vi "Close_Loop_Motor_Tune.vi"() -> ()   [LabVIEW 2019]
uses:
  <vilib>/rvi/Emulation/niFpgaGetClockAttributes.vi
  <vilib>/rvi/Emulation/niFpgaSctlEmulationGetInTimedLoop.vi
  <vilib>/rvi/Emulation/niFpgaEmulationReportErrorSimple.vi
  <vilib>/rvi/eio/common/nirviEmuTemplateMethod_errors.vi
  <vilib>/rvi/Emulation/niFpgaCriticalErrorInLSC.vi
  <vilib>/eio/EIONode/EIONode.xnode
  <vilib>/rvi/Arithmetic/AddSubMult/XNode/nirviSatArithmetic.xnode
panel:
  in  "Motor3_KP":sgl
  in  "Motor2_KP":sgl
  in  "Motor1_KP":sgl=1.2
  in  "Position Reset 3":bool
  out "Position (Counts) motor side 3":i16
  out "Acceleration (Counts/Interval) motor side 3":i32
  out "Velocity (Counts/Interval) motor side 3":i32
  out "Loop time (position) 1 motor side 3":u32
  out "Position(Radians) motor side 3":sgl(graph)
  out "Boolean 4":bool
  in  "desired angle 3":sgl
  in  "Position Reset 2":bool
  out "Position (Counts) motor side 2":i16
  out "Acceleration (Counts/Interval) motor side 2":i32
  out "Velocity (Counts/Interval) motor side 2":i32
  out "Loop time (position) 1 motor side 2":u32
  out "Position(Radians) motor side 2":sgl(graph)
  out "Boolean 3":bool
  in  "desired angle 2":sgl
  in  "Position Reset":bool
  out "Position (Counts) motor side":i16
  out "Acceleration (Counts/Interval) motor side":i32
  out "Velocity (Counts/Interval) motor side":i32
  out "Loop time (position) 1 motor side":u32
  out "Position(Radians) motor side":sgl(graph)
  out "Boolean 2":bool
  in  "desired angle":sgl
  out "duty cycle":sgl
  in  "Position Reset 2_e":bool
  out "Position (Counts) motor side 2_e":i16
  out "Acceleration (Counts/Interval) motor side 2_e":i32
  out "Velocity (Counts/Interval) motor side 2_e":i32
  out "Loop time (position) 1 motor side 2_e":u32
  out "Position(Radians) motor side 2_e":sgl(graph)
  out "Boolean 3_e":bool
  in  "desired angle 2(error)":sgl
  in  "Position Reset 3_e":bool
  out "Position (Counts) motor side 3_e":i16
  out "Acceleration (Counts/Interval) motor side 3_e":i32
  out "Velocity (Counts/Interval) motor side 3_e":i32
  out "Loop time (position) 1 motor side 3_e":u32
  out "Position(Radians) motor side 3_e":sgl(graph)
  out "Boolean 4_e":bool
  in  "desired angle 3(error)":sgl
  in  "Position Reset_e":bool
  out "Position (Counts) motor side_e":i16
  out "Acceleration (Counts/Interval) motor side_e":i32
  out "Velocity (Counts/Interval) motor side_e":i32
  out "Loop time (position) 1 motor side _e":u32
  out "Position(Radians) motor side_e":sgl(graph)
  out "Boolean 2_e":bool
  in  "desired angle (error)":sgl
  out "duty cycle 1_e":sgl
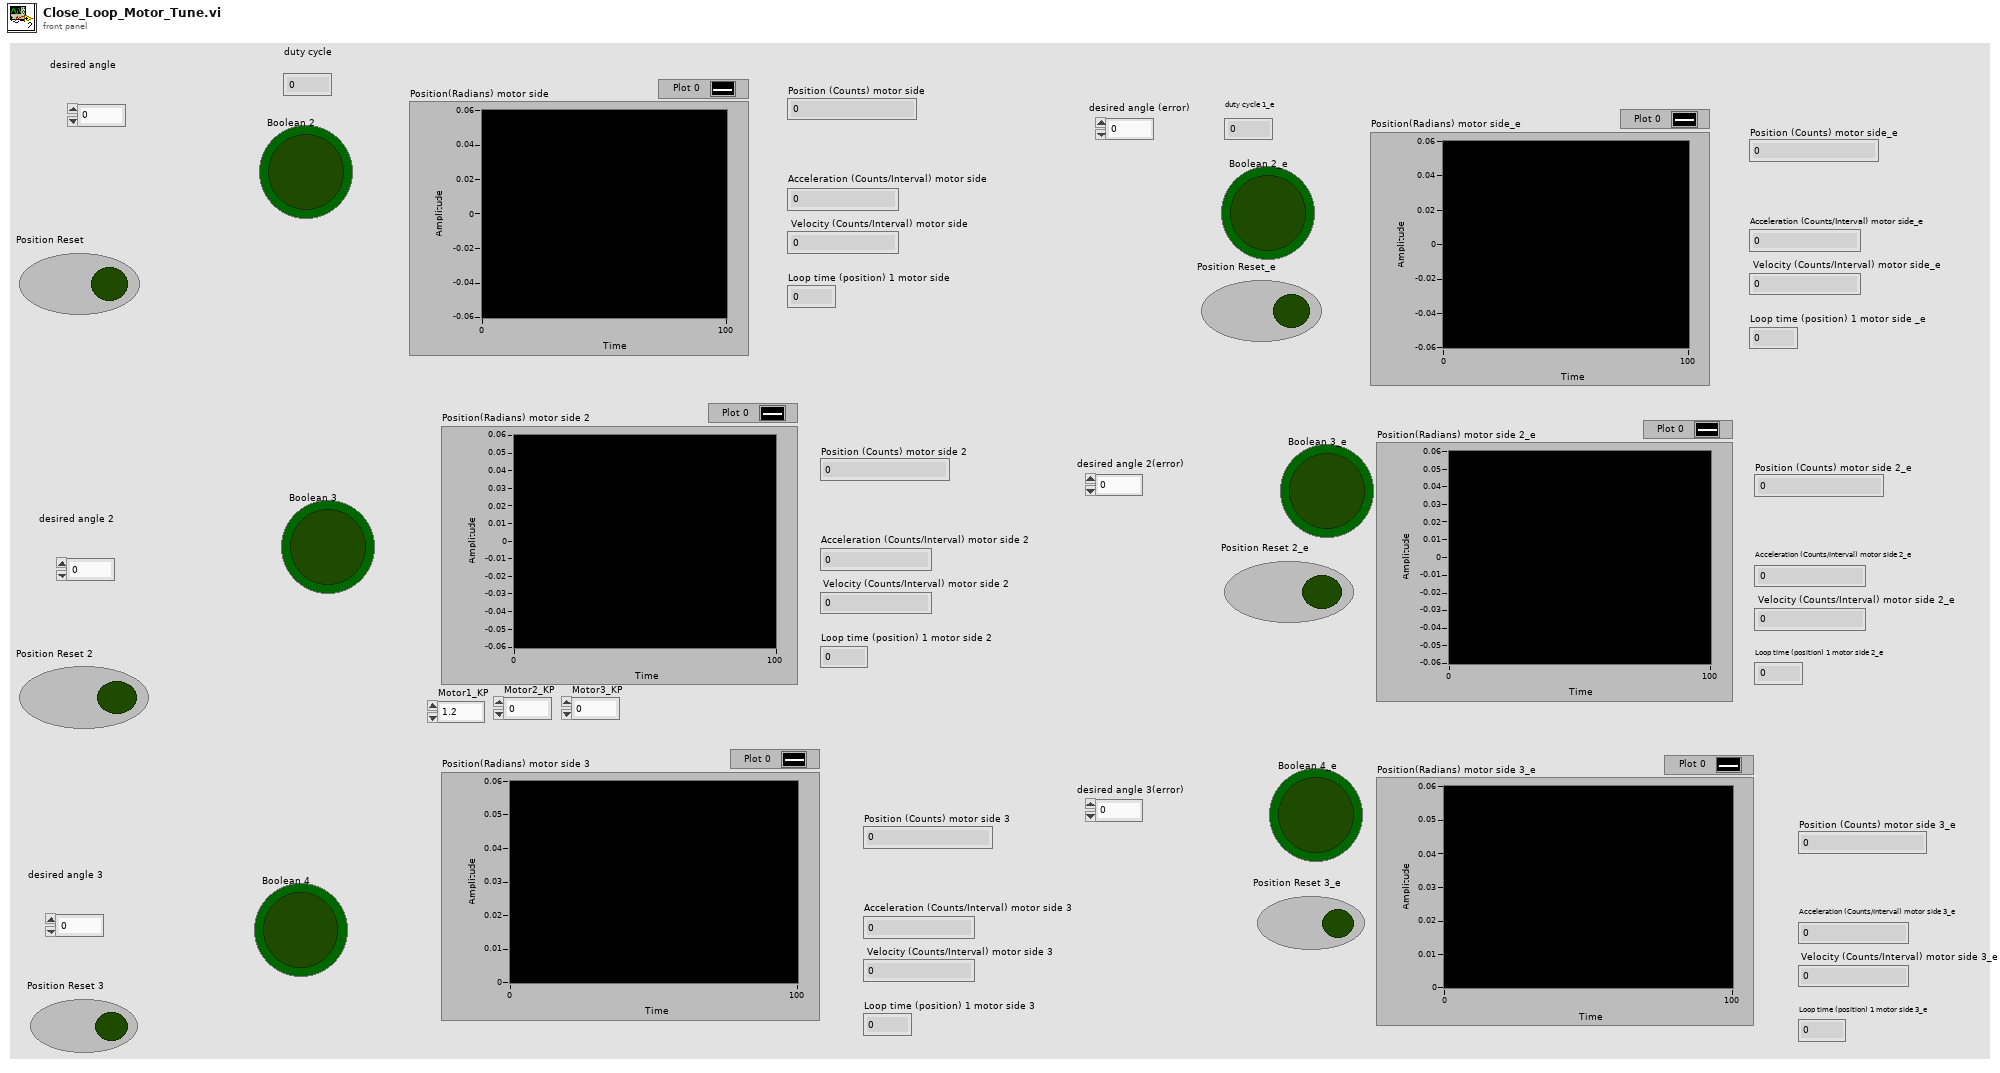
[diagram p1: front panel]
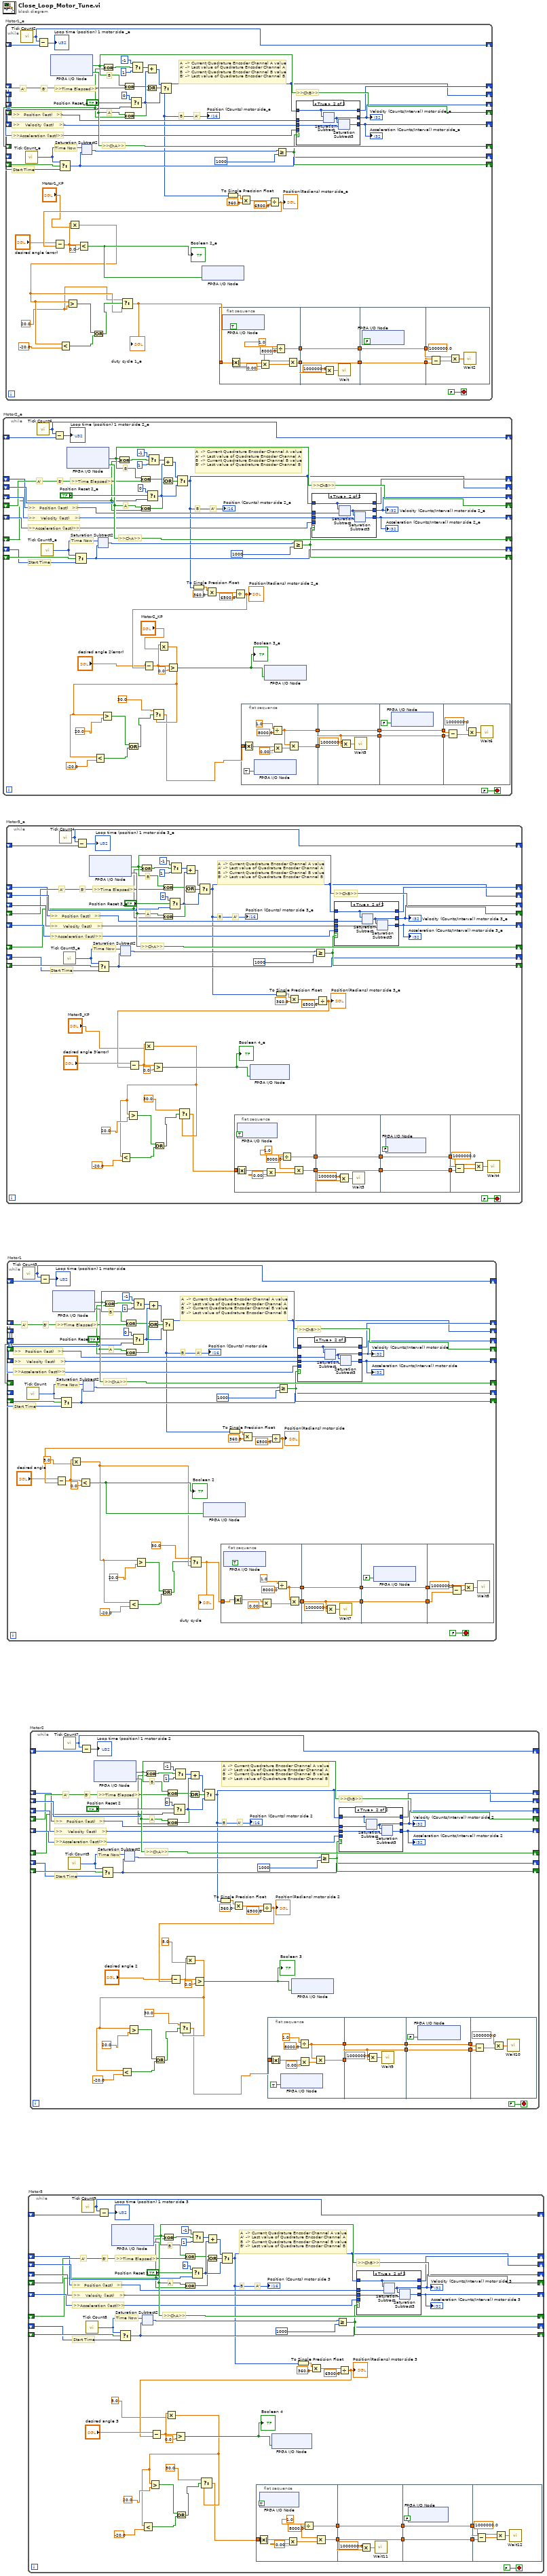
[diagram p0: block diagram]
diagram:
  n1 = while "Motor2_e" {
    shift-right: [w48] -> _
    shift-left: _ -> [w36]
    shift-right: [w28] -> _
    shift-left: _ -> [w45]
    shift-right: [w47] -> _
    shift-left: _ -> [w10]
    shift-right: [w42] -> _
    shift-left: _ -> [w44]
    shift-right: [w38] -> _
    shift-left: _ -> [w43]
    shift-right: [w33] -> _
    shift-left: _ -> [w32]
    shift-right: [w34] -> _
    shift-left: _ -> [w40]
    shift-right: [w35] -> _
    shift-left: _ -> [w37]
    shift-right: [w29] -> _
    shift-left: _ -> [w31]
    stop <- FALSE stop-if-true
    # "A  -> Current Quadrature Encoder Channel A value\nA' -> Last value of Quadrature Encoder Channel A\nB  -> Current Quadrature Encoder Channel B value\nB' -> Last value of Quadrature Encoder Channel B"
    # ">>Acceleration (last)>>"
    # "Start Time"
    # "A'"
    # "B"
    # "A'"
    # "A"
    # "B'"
    # "B"
    # ">>ChB>>"
    # ">>ChA>>"
    # ">>    Velocity (last)    >>"
    # ">>   Position (last)   >>"
    # "Time Now"
    # ">>Time Elapsed>>"
    n2 = call "Tick Count6"() -> ("Tick Count(Ticks)"=w29:u32)
    n3 = call "Tick Count5_e"() -> ("Tick Count(uSec)"=w39:u32)
    n4 = Subtract(x=w29, y=w31) -> (x-y=→"Loop time (position) 1 motor side 2_e":u32)
    n5 = xnode "FPGA I/O Node"() -> ("RMC/DIO12"=w48:bool, "RMC/DIO13"=w47:bool)  [unwired: 2 in, 2 out]
    n6 = Select(t=w39, s=w44, f=w43) -> (s? t:f=w38:u32)
    n7 = xnode ("Saturation Subtract2")("x"=w39, "y"=w38) -> ("x-y"=w41:u32)
    n8 = Exclusive Or(1:w10, 2:w48) -> (0:w49:bool)
    n9 = Exclusive Or(1:w36, 2:w48) -> (0:w50:bool)
    n10 = Exclusive Or(1:w10, 2:w47) -> (0:w51:bool)
    n11 = Select(t=0 ("32 bit"), s="Position Reset 2_e", f=w45) -> (s? t:f=w56:i32)
    n12 = Select(t=-1 ("32 bit"), s=w49, f=1 ("32 bit")) -> (s? t:f=w54:i32)
    n13 = Add(x=w54, y=w56) -> (x+y=w58:i32)
    n14 = Or(x=w50, y=w51) -> (x .or. y?=w46:bool)
    n15 = Select(t=w58, s=w46, f=w56) -> (s? t:f=w28:i32)
    "Position (Counts) motor side 2_e" <- w28
    n16 = To Single Precision Float(number=w28) -> (single precision float=w27:sgl)
    n17 = Multiply(x=w27, y=sgl 360.0) -> (x*y=w26:sgl)
    n18 = Divide(x=w26, y=sgl 6500.0) -> (x/y=w15:sgl)
    "Position(Radians) motor side 2_e" <- w15
    n19 = Subtract(x="desired angle 2(error)", y=w15) -> (x-y=w14:sgl)
    n20 = Multiply(x=w14, y="Motor2_KP") -> (x*y=w3:sgl)
    n21 = Less?(x=w3, y=sgl -20.0) -> (x < y?=w9:bool)
    n22 = Greater?(x=w3, y=sgl 20.0 ("constrain max")) -> (0:w8:bool)
    n23 = Or(x=w8, y=w9) -> (x .or. y?=w5:bool)
    n24 = Select(t=sgl 30.0 ("kp1"), s=w5, f=w3) -> (s? t:f=w2:sgl)
    n25 = Greater?(x=w14, y=sgl 0.0) -> (0:w12:bool)
    "Boolean 3_e" <- w12
    n26 = flat-sequence {
      tunnel: [w64] -> w22
      tunnel: [w62] -> w21
      tunnel: w2 -> [w60]
      tunnel: w22 -> [w69]
      tunnel: [w69] -> w20
      tunnel: w21 -> [w68]
      tunnel: [w68] -> w19
      tunnel: w20 -> [w74]
      tunnel: [w74] -> w18
      tunnel: w19 -> [w73]
      tunnel: [w73] -> w17
      tunnel: w18 -> [w79]
      tunnel: w17 -> [w75]
      frame #0 {
        n27 = Absolute Value(x=w60) -> (abs(x)=w59:sgl)
        n28 = xnode "FPGA I/O Node"("RMC/DIO16"=TRUE) -> ()  [unwired: 1 in, 1 out]
        n29 = Divide(x=sgl 1.0, y=sgl 8000.0) -> (x/y=w62:sgl)
        n30 = Multiply(x=w59, y=sgl 0.01) -> (x*y=w65:sgl)
        n31 = Multiply(x=w62, y=w65) -> (x*y=w64:sgl)
      }
      frame #1 {
        n32 = Multiply(x=sgl 1000000.0, y=w69) -> (x*y=w71:sgl)
        n33 = call "Wait5"("Count(uSec)"=w71) -> ()  [unwired: 1 out]
      }
      frame #2 {
        n34 = xnode "FPGA I/O Node"("RMC/DIO16"=FALSE) -> ()  [unwired: 1 in, 1 out]
      }
      frame #3 {
        n35 = Subtract(x=w75, y=w79) -> (x-y=w78:sgl)
        n36 = Multiply(x=sgl 1000000.0, y=w78) -> (x*y=w77:sgl)
        n37 = call "Wait6"("Count(uSec)"=w77) -> ()  [unwired: 1 out]
      }
    }
    n38 = xnode "FPGA I/O Node"("RMC/DIO17"=w12) -> ()  [unwired: 1 in, 1 out]
    n39 = Greater Or Equal?(x=w41, y=u32 1000) -> (x >= y?=w42:bool)
    n40 = case shown="True" w42 {
      tunnel: w28 -> [_ w93]
      tunnel: w32 -> [w90 w97]
      tunnel: [w92 w96] -> w34
      tunnel: w40 -> [w92 w95]
      tunnel: [w91 w94] -> w35
      tunnel: w37 -> [w91 _]
      tunnel: [w90 w93] -> w33
      frame False {
      }
      frame True {
        n41 = xnode ("Saturation Subtract")("x"=w93, "y"=w97) -> ("x-y"=w96:i32)
        n42 = xnode ("Saturation Subtract3")("x"=w96, "y"=w95) -> ("x-y"=w94:i32)
      }
    }
    "Acceleration (Counts/Interval) motor side 2_e" <- w35
    "Velocity (Counts/Interval) motor side 2_e" <- w34
  }
  n43 = while "Motor1_e" {
    shift-right: [w180] -> _
    shift-left: _ -> [w168]
    shift-right: [w159] -> _
    shift-left: _ -> [w177]
    shift-right: [w179] -> _
    shift-left: _ -> [w160]
    shift-right: [w174] -> _
    shift-left: _ -> [w176]
    shift-right: [w170] -> _
    shift-left: _ -> [w175]
    shift-right: [w165] -> _
    shift-left: _ -> [w164]
    shift-right: [w166] -> _
    shift-left: _ -> [w172]
    shift-right: [w167] -> _
    shift-left: _ -> [w169]
    shift-right: [w161] -> _
    shift-left: _ -> [w163]
    stop <- FALSE stop-if-true
    w136 = sgl 20.0 ("constrain max")
    # "A  -> Current Quadrature Encoder Channel A value\nA' -> Last value of Quadrature Encoder Channel A\nB  -> Current Quadrature Encoder Channel B value\nB' -> Last value of Quadrature Encoder Channel B"
    # ">>Acceleration (last)>>"
    # "Start Time"
    # "A'"
    # "B"
    # "A'"
    # "A"
    # "B'"
    # "B"
    # ">>ChB>>"
    # ">>ChA>>"
    # ">>    Velocity (last)    >>"
    # ">>   Position (last)   >>"
    # "Time Now"
    # ">>Time Elapsed>>"
    n44 = call "Tick Count2"() -> ("Tick Count(Ticks)"=w161:u32)
    n45 = call "Tick Count_e"() -> ("Tick Count(uSec)"=w171:u32)
    n46 = Subtract(x=w161, y=w163) -> (x-y=→"Loop time (position) 1 motor side _e":u32)
    n47 = xnode "FPGA I/O Node"() -> ("RMC/DIO45"=w180:bool, "RMC/DIO43"=w179:bool)  [unwired: 2 in, 2 out]
    n48 = Select(t=w171, s=w176, f=w175) -> (s? t:f=w170:u32)
    n49 = xnode ("Saturation Subtract2")("x"=w171, "y"=w170) -> ("x-y"=w173:u32)
    n50 = Exclusive Or(1:w160, 2:w180) -> (0:w181:bool)
    n51 = Exclusive Or(1:w168, 2:w180) -> (0:w182:bool)
    n52 = Exclusive Or(1:w160, 2:w179) -> (0:w183:bool)
    n53 = Select(t=0 ("32 bit"), s="Position Reset_e", f=w177) -> (s? t:f=w188:i32)
    n54 = Select(t=-1 ("32 bit"), s=w181, f=1 ("32 bit")) -> (s? t:f=w186:i32)
    n55 = Add(x=w186, y=w188) -> (x+y=w190:i32)
    n56 = Or(x=w182, y=w183) -> (x .or. y?=w178:bool)
    n57 = Select(t=w190, s=w178, f=w188) -> (s? t:f=w159:i32)
    "Position (Counts) motor side_e" <- w159
    n58 = flat-sequence {
      tunnel: [w196] -> w153
      tunnel: [w194] -> w152
      tunnel: w138 -> [w192]
      tunnel: w153 -> [w201]
      tunnel: [w201] -> w151
      tunnel: w152 -> [w200]
      tunnel: [w200] -> w150
      tunnel: w151 -> [w206]
      tunnel: [w206] -> w149
      tunnel: w150 -> [w205]
      tunnel: [w205] -> w148
      tunnel: w149 -> [w211]
      tunnel: w148 -> [w207]
      frame #0 {
        n59 = xnode "FPGA I/O Node"("RMC/DIO33"=TRUE) -> ()  [unwired: 1 in, 1 out]
        n60 = Absolute Value(x=w192) -> (abs(x)=w191:sgl)
        n61 = Multiply(x=w191, y=sgl 0.01) -> (x*y=w197:sgl)
        n62 = Divide(x=sgl 1.0, y=sgl 8000.0) -> (x/y=w194:sgl)
        n63 = Multiply(x=w194, y=w197) -> (x*y=w196:sgl)
      }
      frame #1 {
        n64 = Multiply(x=sgl 1000000.0, y=w201) -> (x*y=w203:sgl)
        n65 = call "Wait"("Count(uSec)"=w203) -> ()  [unwired: 1 out]
      }
      frame #2 {
        n66 = xnode "FPGA I/O Node"("RMC/DIO33"=FALSE) -> ()  [unwired: 1 in, 1 out]
      }
      frame #3 {
        n67 = Subtract(x=w207, y=w211) -> (x-y=w210:sgl)
        n68 = Multiply(x=sgl 1000000.0, y=w210) -> (x*y=w209:sgl)
        n69 = call "Wait2"("Count(uSec)"=w209) -> ()  [unwired: 1 out]
      }
    }
    n70 = To Single Precision Float(number=w159) -> (single precision float=w158:sgl)
    n71 = Multiply(x=w158, y=sgl 360.0) -> (x*y=w157:sgl)
    n72 = Divide(x=w157, y=sgl 6500.0) -> (x/y=w146:sgl)
    "Position(Radians) motor side_e" <- w146
    n73 = Subtract(x="desired angle (error)", y=w146) -> (x-y=w144:sgl)
    n74 = Multiply(x=w144, y="Motor1_KP") -> (x*y=w137:sgl)
    n75 = Less?(x=w137, y=sgl -20.0 ("constrain min")) -> (x < y?=w141:bool)
    n76 = Greater?(x=w137, y=w136) -> (0:w140:bool)
    n77 = Less?(x=w144, y=sgl 0.0) -> (x < y?=w143:bool)
    "Boolean 2_e" <- w143
    n78 = Or(x=w140, y=w141) -> (x .or. y?=w139:bool)
    n79 = Select(t=w136, s=w139, f=w137) -> (s? t:f=w138:sgl)
    "duty cycle 1_e" <- w138
    n80 = xnode "FPGA I/O Node"("RMC/DIO34"=w143) -> ()  [unwired: 1 in, 1 out]
    n81 = Greater Or Equal?(x=w173, y=u32 1000) -> (x >= y?=w174:bool)
    n82 = case shown="True" w174 {
      tunnel: w159 -> [_ w225]
      tunnel: w164 -> [w222 w229]
      tunnel: [w224 w228] -> w166
      tunnel: w172 -> [w224 w227]
      tunnel: [w223 w226] -> w167
      tunnel: w169 -> [w223 _]
      tunnel: [w222 w225] -> w165
      frame False {
      }
      frame True {
        n83 = xnode ("Saturation Subtract")("x"=w225, "y"=w229) -> ("x-y"=w228:i32)
        n84 = xnode ("Saturation Subtract3")("x"=w228, "y"=w227) -> ("x-y"=w226:i32)
      }
    }
    "Acceleration (Counts/Interval) motor side_e" <- w167
    "Velocity (Counts/Interval) motor side_e" <- w166
  }
  n85 = while "Motor3_e" {
    shift-right: [w313] -> _
    shift-left: _ -> [w301]
    shift-right: [w292] -> _
    shift-left: _ -> [w310]
    shift-right: [w312] -> _
    shift-left: _ -> [w293]
    shift-right: [w307] -> _
    shift-left: _ -> [w309]
    shift-right: [w303] -> _
    shift-left: _ -> [w308]
    shift-right: [w298] -> _
    shift-left: _ -> [w297]
    shift-right: [w299] -> _
    shift-left: _ -> [w305]
    shift-right: [w300] -> _
    shift-left: _ -> [w302]
    shift-right: [w294] -> _
    shift-left: _ -> [w296]
    stop <- FALSE stop-if-true
    # "A  -> Current Quadrature Encoder Channel A value\nA' -> Last value of Quadrature Encoder Channel A\nB  -> Current Quadrature Encoder Channel B value\nB' -> Last value of Quadrature Encoder Channel B"
    # ">>Acceleration (last)>>"
    # "Start Time"
    # "A'"
    # "B"
    # "A'"
    # "A"
    # "B'"
    # "B"
    # ">>ChB>>"
    # ">>ChA>>"
    # ">>    Velocity (last)    >>"
    # ">>   Position (last)   >>"
    # "Time Now"
    # ">>Time Elapsed>>"
    n86 = call "Tick Count4"() -> ("Tick Count(Ticks)"=w294:u32)
    n87 = call "Tick Count3_e"() -> ("Tick Count(uSec)"=w304:u32)
    n88 = Subtract(x=w294, y=w296) -> (x-y=→"Loop time (position) 1 motor side 3_e":u32)
    n89 = xnode "FPGA I/O Node"() -> ("RMC/DIO11"=w313:bool, "RMC/DIO10"=w312:bool)  [unwired: 2 in, 2 out]
    n90 = Select(t=w304, s=w309, f=w308) -> (s? t:f=w303:u32)
    n91 = xnode ("Saturation Subtract2")("x"=w304, "y"=w303) -> ("x-y"=w306:u32)
    n92 = Exclusive Or(1:w293, 2:w313) -> (0:w314:bool)
    n93 = Exclusive Or(1:w301, 2:w313) -> (0:w315:bool)
    n94 = Exclusive Or(1:w293, 2:w312) -> (0:w316:bool)
    n95 = Select(t=0 ("32 bit"), s="Position Reset 3_e", f=w310) -> (s? t:f=w321:i32)
    n96 = Select(t=-1 ("32 bit"), s=w314, f=1 ("32 bit")) -> (s? t:f=w319:i32)
    n97 = Add(x=w319, y=w321) -> (x+y=w323:i32)
    n98 = Or(x=w315, y=w316) -> (x .or. y?=w311:bool)
    n99 = Select(t=w323, s=w311, f=w321) -> (s? t:f=w292:i32)
    "Position (Counts) motor side 3_e" <- w292
    n100 = flat-sequence {
      tunnel: [w329] -> w286
      tunnel: [w327] -> w285
      tunnel: w268 -> [w325]
      tunnel: w286 -> [w334]
      tunnel: [w334] -> w284
      tunnel: w285 -> [w333]
      tunnel: [w333] -> w283
      tunnel: w284 -> [w339]
      tunnel: [w339] -> w282
      tunnel: w283 -> [w338]
      tunnel: [w338] -> w281
      tunnel: w282 -> [w344]
      tunnel: w281 -> [w340]
      frame #0 {
        n101 = Absolute Value(x=w325) -> (abs(x)=w324:sgl)
        n102 = xnode "FPGA I/O Node"("RMC/DIO0"=TRUE) -> ()  [unwired: 1 in, 1 out]
        n103 = Multiply(x=w324, y=sgl 0.01) -> (x*y=w330:sgl)
        n104 = Divide(x=sgl 1.0, y=sgl 8000.0) -> (x/y=w327:sgl)
        n105 = Multiply(x=w327, y=w330) -> (x*y=w329:sgl)
      }
      frame #1 {
        n106 = Multiply(x=sgl 1000000.0, y=w334) -> (x*y=w336:sgl)
        n107 = call "Wait3"("Count(uSec)"=w336) -> ()  [unwired: 1 out]
      }
      frame #2 {
        n108 = xnode "FPGA I/O Node"("RMC/DIO0"=FALSE) -> ()  [unwired: 1 in, 1 out]
      }
      frame #3 {
        n109 = Subtract(x=w340, y=w344) -> (x-y=w343:sgl)
        n110 = Multiply(x=sgl 1000000.0, y=w343) -> (x*y=w342:sgl)
        n111 = call "Wait4"("Count(uSec)"=w342) -> ()  [unwired: 1 out]
      }
    }
    n112 = To Single Precision Float(number=w292) -> (single precision float=w291:sgl)
    n113 = Multiply(x=w291, y=sgl 360.0) -> (x*y=w290:sgl)
    n114 = Greater Or Equal?(x=w306, y=u32 1000) -> (x >= y?=w307:bool)
    n115 = Divide(x=w290, y=sgl 6500.0) -> (x/y=w278:sgl)
    "Position(Radians) motor side 3_e" <- w278
    n116 = Subtract(x="desired angle 3(error)", y=w278) -> (x-y=w277:sgl)
    n117 = Multiply(x=w277, y="Motor3_KP") -> (x*y=w269:sgl)
    n118 = Less?(x=w269, y=sgl -20.0) -> (x < y?=w274:bool)
    n119 = Greater?(x=w269, y=sgl 20.0 ("constrain max")) -> (0:w273:bool)
    n120 = Greater?(x=w277, y=sgl 0.0) -> (0:w275:bool)
    "Boolean 4_e" <- w275
    n121 = Or(x=w273, y=w274) -> (x .or. y?=w270:bool)
    n122 = Select(t=sgl 30.0 ("kp1"), s=w270, f=w269) -> (s? t:f=w268:sgl)
    n123 = xnode "FPGA I/O Node"("RMC/DIO1"=w275) -> ()  [unwired: 1 in, 1 out]
    n124 = case shown="True" w307 {
      tunnel: w292 -> [_ w358]
      tunnel: w297 -> [w355 w362]
      tunnel: [w357 w361] -> w299
      tunnel: w305 -> [w357 w360]
      tunnel: [w356 w359] -> w300
      tunnel: w302 -> [w356 _]
      tunnel: [w355 w358] -> w298
      frame False {
      }
      frame True {
        n125 = xnode ("Saturation Subtract")("x"=w358, "y"=w362) -> ("x-y"=w361:i32)
        n126 = xnode ("Saturation Subtract3")("x"=w361, "y"=w360) -> ("x-y"=w359:i32)
      }
    }
    "Acceleration (Counts/Interval) motor side 3_e" <- w300
    "Velocity (Counts/Interval) motor side 3_e" <- w299
  }
  n127 = while "Motor1" {
    shift-right: [w446] -> _
    shift-left: _ -> [w434]
    shift-right: [w425] -> _
    shift-left: _ -> [w443]
    shift-right: [w445] -> _
    shift-left: _ -> [w426]
    shift-right: [w440] -> _
    shift-left: _ -> [w442]
    shift-right: [w436] -> _
    shift-left: _ -> [w441]
    shift-right: [w431] -> _
    shift-left: _ -> [w430]
    shift-right: [w432] -> _
    shift-left: _ -> [w438]
    shift-right: [w433] -> _
    shift-left: _ -> [w435]
    shift-right: [w427] -> _
    shift-left: _ -> [w429]
    stop <- FALSE stop-if-true
    # "A  -> Current Quadrature Encoder Channel A value\nA' -> Last value of Quadrature Encoder Channel A\nB  -> Current Quadrature Encoder Channel B value\nB' -> Last value of Quadrature Encoder Channel B"
    # ">>Acceleration (last)>>"
    # "Start Time"
    # "A'"
    # "B"
    # "A'"
    # "A"
    # "B'"
    # "B"
    # ">>ChB>>"
    # ">>ChA>>"
    # ">>    Velocity (last)    >>"
    # ">>   Position (last)   >>"
    # "Time Now"
    # ">>Time Elapsed>>"
    n128 = call "Tick Count3"() -> ("Tick Count(Ticks)"=w427:u32)
    n129 = call "Tick Count"() -> ("Tick Count(uSec)"=w437:u32)
    n130 = Subtract(x=w427, y=w429) -> (x-y=→"Loop time (position) 1 motor side":u32)
    n131 = xnode "FPGA I/O Node"() -> ("RMC/DIO45"=w446:bool, "RMC/DIO43"=w445:bool)  [unwired: 2 in, 2 out]
    n132 = Select(t=w437, s=w442, f=w441) -> (s? t:f=w436:u32)
    n133 = xnode ("Saturation Subtract2")("x"=w437, "y"=w436) -> ("x-y"=w439:u32)
    n134 = Exclusive Or(1:w426, 2:w446) -> (0:w447:bool)
    n135 = Exclusive Or(1:w434, 2:w446) -> (0:w448:bool)
    n136 = Exclusive Or(1:w426, 2:w445) -> (0:w449:bool)
    n137 = Select(t=0 ("32 bit"), s="Position Reset", f=w443) -> (s? t:f=w454:i32)
    n138 = Select(t=-1 ("32 bit"), s=w447, f=1 ("32 bit")) -> (s? t:f=w452:i32)
    n139 = Add(x=w452, y=w454) -> (x+y=w456:i32)
    n140 = Or(x=w448, y=w449) -> (x .or. y?=w444:bool)
    n141 = Select(t=w456, s=w444, f=w454) -> (s? t:f=w425:i32)
    "Position (Counts) motor side" <- w425
    n142 = flat-sequence {
      tunnel: [w462] -> w419
      tunnel: [w460] -> w418
      tunnel: w405 -> [w458]
      tunnel: w419 -> [w467]
      tunnel: [w467] -> w417
      tunnel: w418 -> [w466]
      tunnel: [w466] -> w416
      tunnel: w417 -> [w472]
      tunnel: [w472] -> w415
      tunnel: w416 -> [w471]
      tunnel: [w471] -> w414
      tunnel: w415 -> [w477]
      tunnel: w414 -> [w473]
      frame #0 {
        n143 = xnode "FPGA I/O Node"("RMC/DIO33"=TRUE) -> ()  [unwired: 1 in, 1 out]
        n144 = Absolute Value(x=w458) -> (abs(x)=w457:sgl)
        n145 = Multiply(x=w457, y=sgl 0.01) -> (x*y=w463:sgl)
        n146 = Divide(x=sgl 1.0, y=sgl 8000.0) -> (x/y=w460:sgl)
        n147 = Multiply(x=w460, y=w463) -> (x*y=w462:sgl)
      }
      frame #1 {
        n148 = Multiply(x=sgl 1000000.0, y=w467) -> (x*y=w469:sgl)
        n149 = call "Wait7"("Count(uSec)"=w469) -> ()  [unwired: 1 out]
      }
      frame #2 {
        n150 = xnode "FPGA I/O Node"("RMC/DIO33"=FALSE) -> ()  [unwired: 1 in, 1 out]
      }
      frame #3 {
        n151 = Subtract(x=w473, y=w477) -> (x-y=w476:sgl)
        n152 = Multiply(x=sgl 1000000.0, y=w476) -> (x*y=w475:sgl)
        n153 = call "Wait8"("Count(uSec)"=w475) -> ()  [unwired: 1 out]
      }
    }
    n154 = To Single Precision Float(number=w425) -> (single precision float=w424:sgl)
    n155 = Multiply(x=w424, y=sgl 360.0) -> (x*y=w423:sgl)
    n156 = Divide(x=w423, y=sgl 6500.0) -> (x/y=w412:sgl)
    "Position(Radians) motor side" <- w412
    n157 = Subtract(x="desired angle", y=w412) -> (x-y=w410:sgl)
    n158 = Multiply(x=w410, y=sgl 5.0 ("kp1")) -> (x*y=w404:sgl)
    n159 = Less?(x=w410, y=sgl 0.0) -> (x < y?=w409:bool)
    "Boolean 2" <- w409
    n160 = Less?(x=w404, y=sgl -20.0) -> (x < y?=w403:bool)
    n161 = Greater?(x=w404, y=sgl 20.0 ("constrain max")) -> (0:w402:bool)
    n162 = Or(x=w402, y=w403) -> (x .or. y?=w401:bool)
    n163 = Select(t=sgl 30.0 ("kp1"), s=w401, f=w404) -> (s? t:f=w405:sgl)
    "duty cycle" <- w405
    n164 = xnode "FPGA I/O Node"("RMC/DIO34"=w409) -> ()  [unwired: 1 in, 1 out]
    n165 = Greater Or Equal?(x=w439, y=u32 1000) -> (x >= y?=w440:bool)
    n166 = case shown="True" w440 {
      tunnel: w425 -> [_ w491]
      tunnel: w430 -> [w488 w495]
      tunnel: [w490 w494] -> w432
      tunnel: w438 -> [w490 w493]
      tunnel: [w489 w492] -> w433
      tunnel: w435 -> [w489 _]
      tunnel: [w488 w491] -> w431
      frame False {
      }
      frame True {
        n167 = xnode ("Saturation Subtract")("x"=w491, "y"=w495) -> ("x-y"=w494:i32)
        n168 = xnode ("Saturation Subtract3")("x"=w494, "y"=w493) -> ("x-y"=w492:i32)
      }
    }
    "Acceleration (Counts/Interval) motor side" <- w433
    "Velocity (Counts/Interval) motor side" <- w432
  }
  n169 = while "Motor3" {
    shift-right: [w579] -> _
    shift-left: _ -> [w567]
    shift-right: [w558] -> _
    shift-left: _ -> [w576]
    shift-right: [w578] -> _
    shift-left: _ -> [w559]
    shift-right: [w573] -> _
    shift-left: _ -> [w575]
    shift-right: [w569] -> _
    shift-left: _ -> [w574]
    shift-right: [w564] -> _
    shift-left: _ -> [w563]
    shift-right: [w565] -> _
    shift-left: _ -> [w571]
    shift-right: [w566] -> _
    shift-left: _ -> [w568]
    shift-right: [w560] -> _
    shift-left: _ -> [w562]
    stop <- FALSE stop-if-true
    # "A  -> Current Quadrature Encoder Channel A value\nA' -> Last value of Quadrature Encoder Channel A\nB  -> Current Quadrature Encoder Channel B value\nB' -> Last value of Quadrature Encoder Channel B"
    # ">>Acceleration (last)>>"
    # "Start Time"
    # "A'"
    # "B"
    # "A'"
    # "A"
    # "B'"
    # "B"
    # ">>ChB>>"
    # ">>ChA>>"
    # ">>    Velocity (last)    >>"
    # ">>   Position (last)   >>"
    # "Time Now"
    # ">>Time Elapsed>>"
    n170 = call "Tick Count9"() -> ("Tick Count(Ticks)"=w560:u32)
    n171 = call "Tick Count8"() -> ("Tick Count(uSec)"=w570:u32)
    n172 = Subtract(x=w560, y=w562) -> (x-y=→"Loop time (position) 1 motor side 3":u32)
    n173 = xnode "FPGA I/O Node"() -> ("RMC/DIO11"=w579:bool, "RMC/DIO10"=w578:bool)  [unwired: 2 in, 2 out]
    n174 = Select(t=w570, s=w575, f=w574) -> (s? t:f=w569:u32)
    n175 = xnode ("Saturation Subtract2")("x"=w570, "y"=w569) -> ("x-y"=w572:u32)
    n176 = Exclusive Or(1:w559, 2:w579) -> (0:w580:bool)
    n177 = Exclusive Or(1:w567, 2:w579) -> (0:w581:bool)
    n178 = Exclusive Or(1:w559, 2:w578) -> (0:w582:bool)
    n179 = Select(t=0 ("32 bit"), s="Position Reset 3", f=w576) -> (s? t:f=w587:i32)
    n180 = Select(t=-1 ("32 bit"), s=w580, f=1 ("32 bit")) -> (s? t:f=w585:i32)
    n181 = Add(x=w585, y=w587) -> (x+y=w589:i32)
    n182 = Or(x=w581, y=w582) -> (x .or. y?=w577:bool)
    n183 = Select(t=w589, s=w577, f=w587) -> (s? t:f=w558:i32)
    "Position (Counts) motor side 3" <- w558
    n184 = flat-sequence {
      tunnel: [w595] -> w552
      tunnel: [w593] -> w551
      tunnel: w533 -> [w591]
      tunnel: w552 -> [w600]
      tunnel: [w600] -> w550
      tunnel: w551 -> [w599]
      tunnel: [w599] -> w549
      tunnel: w550 -> [w605]
      tunnel: [w605] -> w548
      tunnel: w549 -> [w604]
      tunnel: [w604] -> w547
      tunnel: w548 -> [w610]
      tunnel: w547 -> [w606]
      frame #0 {
        n185 = Absolute Value(x=w591) -> (abs(x)=w590:sgl)
        n186 = xnode "FPGA I/O Node"("RMC/DIO0"=TRUE) -> ()  [unwired: 1 in, 1 out]
        n187 = Multiply(x=w590, y=sgl 0.01) -> (x*y=w596:sgl)
        n188 = Divide(x=sgl 1.0, y=sgl 8000.0) -> (x/y=w593:sgl)
        n189 = Multiply(x=w593, y=w596) -> (x*y=w595:sgl)
      }
      frame #1 {
        n190 = Multiply(x=sgl 1000000.0, y=w600) -> (x*y=w602:sgl)
        n191 = call "Wait11"("Count(uSec)"=w602) -> ()  [unwired: 1 out]
      }
      frame #2 {
        n192 = xnode "FPGA I/O Node"("RMC/DIO0"=FALSE) -> ()  [unwired: 1 in, 1 out]
      }
      frame #3 {
        n193 = Subtract(x=w606, y=w610) -> (x-y=w609:sgl)
        n194 = Multiply(x=sgl 1000000.0, y=w609) -> (x*y=w608:sgl)
        n195 = call "Wait12"("Count(uSec)"=w608) -> ()  [unwired: 1 out]
      }
    }
    n196 = To Single Precision Float(number=w558) -> (single precision float=w557:sgl)
    n197 = Multiply(x=w557, y=sgl 360.0) -> (x*y=w556:sgl)
    n198 = Greater Or Equal?(x=w572, y=u32 1000) -> (x >= y?=w573:bool)
    n199 = Divide(x=w556, y=sgl 6500.0) -> (x/y=w544:sgl)
    "Position(Radians) motor side 3" <- w544
    n200 = Subtract(x="desired angle 3", y=w544) -> (x-y=w543:sgl)
    n201 = Multiply(x=w543, y=sgl 5.0) -> (x*y=w534:sgl)
    n202 = Less?(x=w534, y=sgl -20.0) -> (x < y?=w539:bool)
    n203 = Greater?(x=w534, y=sgl 20.0 ("constrain max")) -> (0:w538:bool)
    n204 = Greater?(x=w543, y=sgl 0.0) -> (0:w541:bool)
    "Boolean 4" <- w541
    n205 = Or(x=w538, y=w539) -> (x .or. y?=w535:bool)
    n206 = Select(t=sgl 30.0 ("kp1"), s=w535, f=w534) -> (s? t:f=w533:sgl)
    n207 = xnode "FPGA I/O Node"("RMC/DIO1"=w541) -> ()  [unwired: 1 in, 1 out]
    n208 = case shown="True" w573 {
      tunnel: w558 -> [_ w624]
      tunnel: w563 -> [w621 w628]
      tunnel: [w623 w627] -> w565
      tunnel: w571 -> [w623 w626]
      tunnel: [w622 w625] -> w566
      tunnel: w568 -> [w622 _]
      tunnel: [w621 w624] -> w564
      frame False {
      }
      frame True {
        n209 = xnode ("Saturation Subtract")("x"=w624, "y"=w628) -> ("x-y"=w627:i32)
        n210 = xnode ("Saturation Subtract3")("x"=w627, "y"=w626) -> ("x-y"=w625:i32)
      }
    }
    "Acceleration (Counts/Interval) motor side 3" <- w566
    "Velocity (Counts/Interval) motor side 3" <- w565
  }
  n211 = while "Motor2" {
    shift-right: [w712] -> _
    shift-left: _ -> [w700]
    shift-right: [w692] -> _
    shift-left: _ -> [w709]
    shift-right: [w711] -> _
    shift-left: _ -> [w673]
    shift-right: [w706] -> _
    shift-left: _ -> [w708]
    shift-right: [w702] -> _
    shift-left: _ -> [w707]
    shift-right: [w697] -> _
    shift-left: _ -> [w696]
    shift-right: [w698] -> _
    shift-left: _ -> [w704]
    shift-right: [w699] -> _
    shift-left: _ -> [w701]
    shift-right: [w693] -> _
    shift-left: _ -> [w695]
    stop <- FALSE stop-if-true
    # "A  -> Current Quadrature Encoder Channel A value\nA' -> Last value of Quadrature Encoder Channel A\nB  -> Current Quadrature Encoder Channel B value\nB' -> Last value of Quadrature Encoder Channel B"
    # ">>Acceleration (last)>>"
    # "Start Time"
    # "A'"
    # "B"
    # "A'"
    # "A"
    # "B'"
    # "B"
    # ">>ChB>>"
    # ">>ChA>>"
    # ">>    Velocity (last)    >>"
    # ">>   Position (last)   >>"
    # "Time Now"
    # ">>Time Elapsed>>"
    n212 = call "Tick Count7"() -> ("Tick Count(Ticks)"=w693:u32)
    n213 = call "Tick Count5"() -> ("Tick Count(uSec)"=w703:u32)
    n214 = Subtract(x=w693, y=w695) -> (x-y=→"Loop time (position) 1 motor side 2":u32)
    n215 = xnode "FPGA I/O Node"() -> ("RMC/DIO12"=w712:bool, "RMC/DIO13"=w711:bool)  [unwired: 2 in, 2 out]
    n216 = Select(t=w703, s=w708, f=w707) -> (s? t:f=w702:u32)
    n217 = xnode ("Saturation Subtract2")("x"=w703, "y"=w702) -> ("x-y"=w705:u32)
    n218 = Exclusive Or(1:w673, 2:w712) -> (0:w713:bool)
    n219 = Exclusive Or(1:w700, 2:w712) -> (0:w714:bool)
    n220 = Exclusive Or(1:w673, 2:w711) -> (0:w715:bool)
    n221 = Select(t=0 ("32 bit"), s="Position Reset 2", f=w709) -> (s? t:f=w720:i32)
    n222 = Select(t=-1 ("32 bit"), s=w713, f=1 ("32 bit")) -> (s? t:f=w718:i32)
    n223 = Add(x=w718, y=w720) -> (x+y=w722:i32)
    n224 = Or(x=w714, y=w715) -> (x .or. y?=w710:bool)
    n225 = Select(t=w722, s=w710, f=w720) -> (s? t:f=w692:i32)
    "Position (Counts) motor side 2" <- w692
    n226 = To Single Precision Float(number=w692) -> (single precision float=w691:sgl)
    n227 = Multiply(x=w691, y=sgl 360.0) -> (x*y=w690:sgl)
    n228 = Divide(x=w690, y=sgl 6500.0) -> (x/y=w679:sgl)
    "Position(Radians) motor side 2" <- w679
    n229 = Subtract(x="desired angle 2", y=w679) -> (x-y=w678:sgl)
    n230 = Multiply(x=w678, y=sgl 5.0) -> (x*y=w666:sgl)
    n231 = Less?(x=w666, y=sgl -20.0) -> (x < y?=w672:bool)
    n232 = Greater?(x=w666, y=sgl 20.0 ("constrain max")) -> (0:w671:bool)
    n233 = Or(x=w671, y=w672) -> (x .or. y?=w668:bool)
    n234 = Select(t=sgl 30.0 ("kp1"), s=w668, f=w666) -> (s? t:f=w665:sgl)
    n235 = Greater?(x=w678, y=sgl 0.0) -> (0:w676:bool)
    "Boolean 3" <- w676
    n236 = flat-sequence {
      tunnel: [w728] -> w686
      tunnel: [w726] -> w685
      tunnel: w665 -> [w724]
      tunnel: w686 -> [w733]
      tunnel: [w733] -> w684
      tunnel: w685 -> [w732]
      tunnel: [w732] -> w683
      tunnel: w684 -> [w738]
      tunnel: [w738] -> w682
      tunnel: w683 -> [w737]
      tunnel: [w737] -> w681
      tunnel: w682 -> [w743]
      tunnel: w681 -> [w739]
      frame #0 {
        n237 = Absolute Value(x=w724) -> (abs(x)=w723:sgl)
        n238 = xnode "FPGA I/O Node"("RMC/DIO16"=TRUE) -> ()  [unwired: 1 in, 1 out]
        n239 = Divide(x=sgl 1.0, y=sgl 8000.0) -> (x/y=w726:sgl)
        n240 = Multiply(x=w723, y=sgl 0.01) -> (x*y=w729:sgl)
        n241 = Multiply(x=w726, y=w729) -> (x*y=w728:sgl)
      }
      frame #1 {
        n242 = Multiply(x=sgl 1000000.0, y=w733) -> (x*y=w735:sgl)
        n243 = call "Wait9"("Count(uSec)"=w735) -> ()  [unwired: 1 out]
      }
      frame #2 {
        n244 = xnode "FPGA I/O Node"("RMC/DIO16"=FALSE) -> ()  [unwired: 1 in, 1 out]
      }
      frame #3 {
        n245 = Subtract(x=w739, y=w743) -> (x-y=w742:sgl)
        n246 = Multiply(x=sgl 1000000.0, y=w742) -> (x*y=w741:sgl)
        n247 = call "Wait10"("Count(uSec)"=w741) -> ()  [unwired: 1 out]
      }
    }
    n248 = xnode "FPGA I/O Node"("RMC/DIO17"=w676) -> ()  [unwired: 1 in, 1 out]
    n249 = Greater Or Equal?(x=w705, y=u32 1000) -> (x >= y?=w706:bool)
    n250 = case shown="True" w706 {
      tunnel: w692 -> [_ w757]
      tunnel: w696 -> [w754 w761]
      tunnel: [w756 w760] -> w698
      tunnel: w704 -> [w756 w759]
      tunnel: [w755 w758] -> w699
      tunnel: w701 -> [w755 _]
      tunnel: [w754 w757] -> w697
      frame False {
      }
      frame True {
        n251 = xnode ("Saturation Subtract")("x"=w757, "y"=w761) -> ("x-y"=w760:i32)
        n252 = xnode ("Saturation Subtract3")("x"=w760, "y"=w759) -> ("x-y"=w758:i32)
      }
    }
    "Acceleration (Counts/Interval) motor side 2" <- w699
    "Velocity (Counts/Interval) motor side 2" <- w698
  }
